vi "Str_range.vi"(9 "step":sgl=5e-10 format="%#_6p", 10 "end":sgl=5e-10 format="%#_6p", 11 "start":sgl=5e-10 format="%#_6p") -> (3 "Item Names":string[](array[string]))   [LabVIEW 2014]
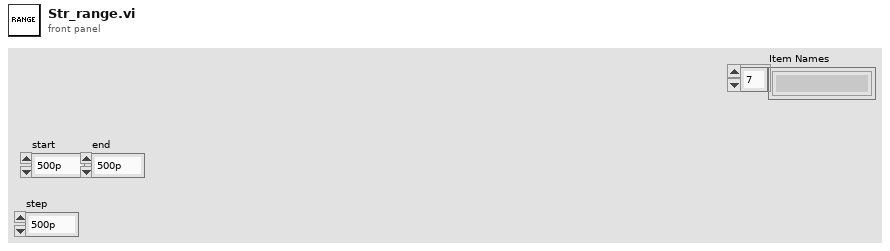
[diagram p1: front panel]
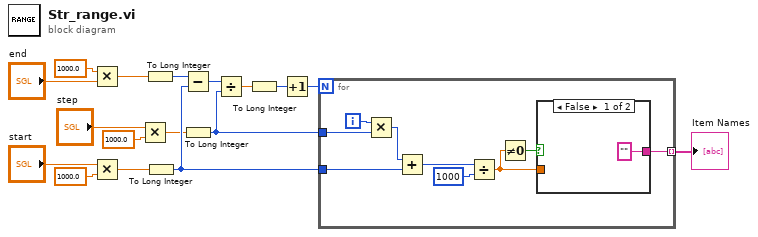
[diagram p0: block diagram]
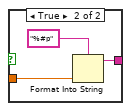
[diagram p2: hidden frame]
diagram:
  n1 = Multiply(x=sgl 1000.0, y="end") -> (x*y=w12:sgl)
  n2 = Multiply(x="start", y=sgl 1000.0) -> (x*y=w9:sgl)
  n3 = Multiply(x="step", y=sgl 1000.0) -> (x*y=w5:sgl)
  n4 = To Long Integer(number=w12) -> (32bit integer=w10:i32)
  n5 = To Long Integer(number=w9) -> (32bit integer=w6:i32)
  n6 = Subtract(x=w10, y=w6) -> (x-y=w14:i32)
  n7 = To Long Integer(number=w5) -> (32bit integer=w2:i32)
  n8 = Divide(x=w14, y=w2) -> (x/y=w13:dbl)
  n9 = To Long Integer(number=w13) -> (32bit integer=w15:i32)
  n10 = Increment(x=w15) -> (x+1=w1:i32)
  n11 = for {
    N: w1 -> [_]
    tunnel: w6 -> [w26]
    tunnel: w2 -> [w25]
    tunnel: [w22] -> w17 mode=indexing
    i -> [w23]
    n12 = Multiply(x=w23, y=w25) -> (x*y=w24:i32)
    n13 = Add(x=w24, y=w26) -> (x+y=w21:i32)
    n14 = Divide(x=w21, y=1000) -> (x/y=w18:dbl)
    n15 = Not Equal To 0?(x=w18) -> (x != 0?=w19:bool)
    n16 = case shown="False" w19 {
      tunnel: ["" w29] -> w22
      tunnel: w18 -> [_ w28]
      frame False {
      }
      frame True {
        n17 = Format Into String(format string="%#p", w28) -> (resulting string=w29:string)  [unwired: 2 in, 1 out]
      }
    }
  }
  "Item Names" <- w17
